vi "IMU Get Yaw Portrait.vi"(8 "error in (no error)":errorcluster) -> (0 "error out":errorcluster, 2 "timestamp out":i64, 3 "yaw":dbl(graph))   [LabVIEW 2026, in "MrcLib.lvlib"]
doc: "Return the computed Yaw of the built-in sensor assuming the controller is mounted vertical with narrow edge parallel to the ground (less common)."
uses:
  MrcLib.lvlib
panel:
  out "yaw out":dbl
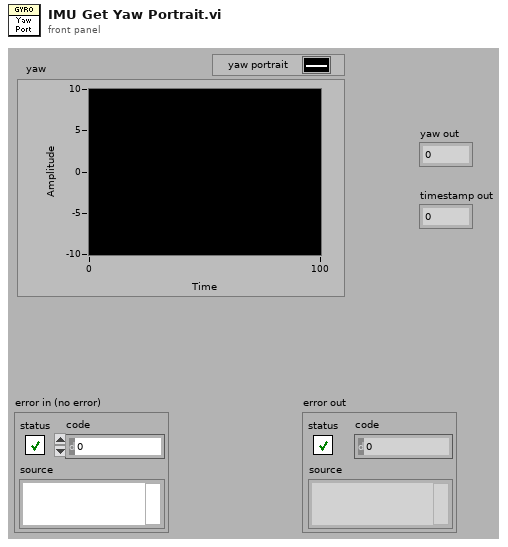
[diagram p1: front panel]
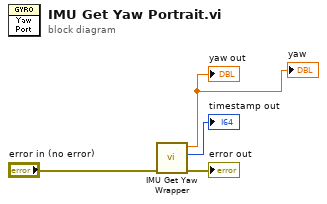
[diagram p0: block diagram]
diagram:
  n1 = call-poly "IMU Get Yaw Wrapper.vi"("error in (no error)"="error in (no error)") -> ("error out"=→"error out":errorcluster, "timestamp out"=→"timestamp out":i64, "yaw out"=→"yaw out" →"yaw":dbl)  [unwired: 7 in, 1 out]
